vi "XSP3_SetFileNumber.vi"(6 "Number":i32 caption="FileNumber", 8 "ErrorIn":errorcluster, 11 "ProcessIn":string="XSPRESS3-EXAMPLE" caption="ProcessName") -> (0 "ErrorOut":errorcluster, 2 "Status":bool, 3 "ProcessOut":string caption="ProcessName")   [LabVIEW 2010]
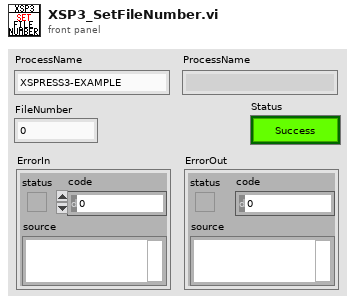
[diagram p1: front panel]
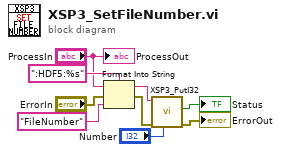
[diagram p0: block diagram]
diagram:
  n1 = Format Into String(format string=":HDF5:%s" ("PV"), initial string="ProcessIn", error in="ErrorIn", "FileNumber" ("PV")) -> (resulting string=w1:string, error out=w2:errorcluster)
  n2 = call "XSP3_PutI32.vi"("I32"="Number", "ErrorIn"=w2, "PVIn"=w1) -> ("ErrorOut"=→"ErrorOut":errorcluster, "Status"=→"Status":bool)  [unwired: 5 in, 2 out]
  "ProcessOut" <- "ProcessIn"
